vi "Filter_Where.vi"(11 "Filter In":T1[](array[typedef])) -> (3 "WHERE?":string)   [LabVIEW 2020]
uses:
  Controls/Filter.ctl
  Controls/Comparator.ctl
panel:
  out "Array":string[](array[string])
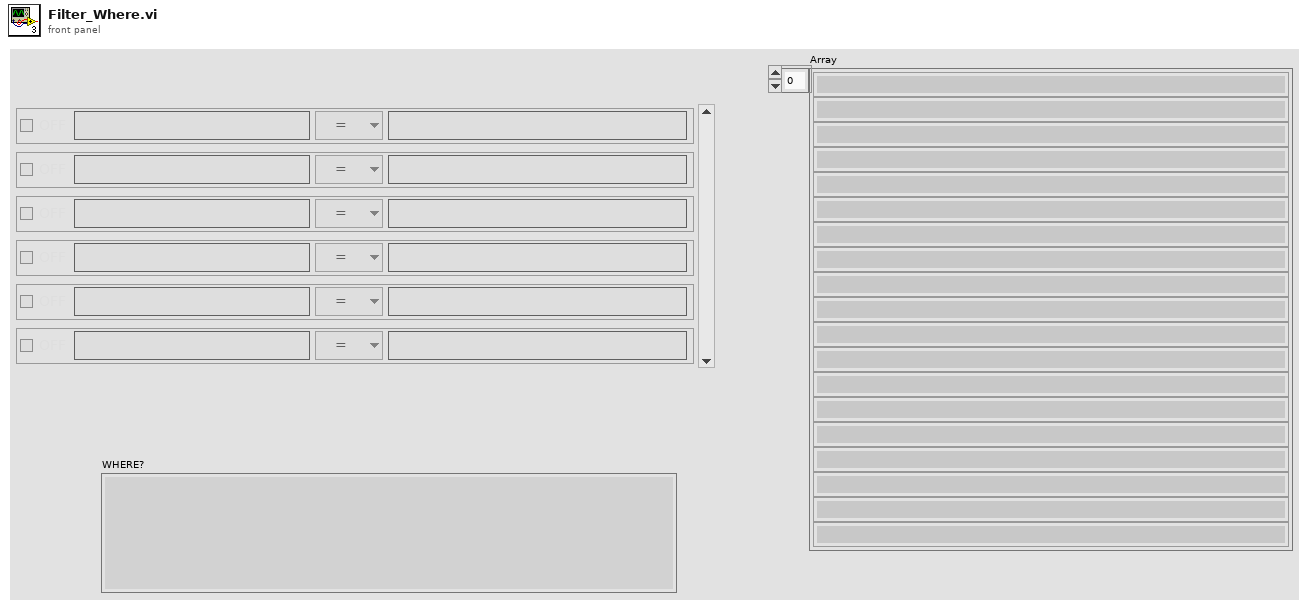
[diagram p1: front panel]
types:
  T1 = typedef "Filter.ctl" = cluster{"Select":bool, "Column":string, "Compare":T2, "Data":string}
  T2 = typedef "Comparator.ctl" = enum16{"=", "<=", ">=", "<", ">", "Like"}
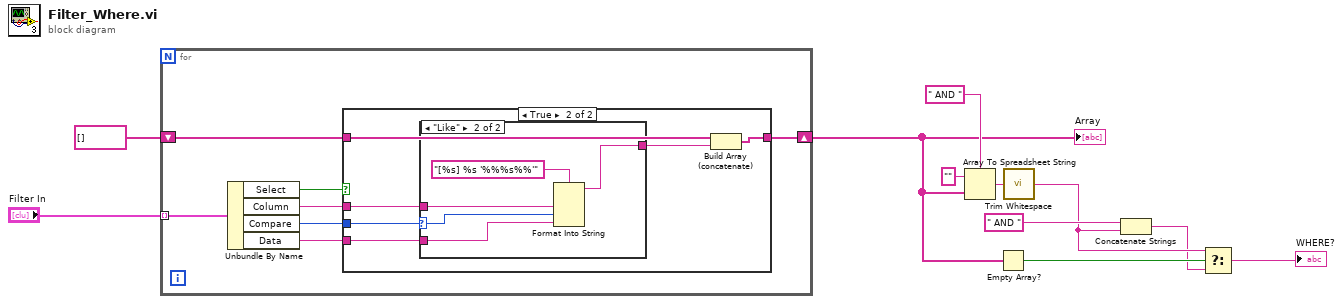
[diagram p0: block diagram]
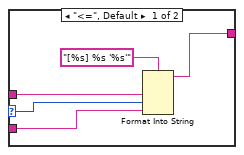
[diagram p3: hidden frame]
diagram:
  n1 = for {
    tunnel: "Filter In" -> [w18] mode=indexing
    shift-right: [w12] -> w6
    shift-left: string[] [] -> [w13]
    n2 = Unbundle By Name(w18) -> ("Select"=w17:bool, "Column"=w16:string, "Compare"=w15:T2, "Data"=w14:string)
    n3 = case shown="True" w17 {
      tunnel: w16 -> [_ w25]
      tunnel: w15 -> [_ w20]
      tunnel: w14 -> [_ w24]
      tunnel: w13 -> [w19 w23]
      tunnel: [w19 w21] -> w12
      frame False {
      }
      frame True {
        n4 = case shown="\"Like\"" w20 {
          selector: w20 -> [w26 w31]
          tunnel: w25 -> [w29 w34]
          tunnel: w24 -> [w28 w33]
          tunnel: [w27 w32] -> w22
          frame "<=", Default {
            n5 = Format Into String(format string="[%s] %s '%s'", w29, w26, w28) -> (resulting string=w27:string)  [unwired: 2 in, 1 out]
          }
          frame "Like" {
            n6 = Format Into String(format string="[%s] %s '%%%s%%'", w34, w31, w33) -> (resulting string=w32:string)  [unwired: 2 in, 1 out]
          }
        }
        n7 = Build Array (concatenate)(w23, w22) -> (w21:string[])
      }
    }
  }
  "Array" <- w6
  n8 = Array To Spreadsheet String(delimiter (Tab)=" AND ", array=w6, 3:"" ("format string")) -> (spreadsheet string=w7:string)
  n9 = Empty Array?(array=w6) -> (empty?=w5:bool)
  n10 = call <vilib>:"Trim Whitespace.vi"("string"=w7) -> ("trimmed string"=w2:string)  [unwired: 1 in]
  n11 = Concatenate Strings(" AND " ("string"), w2) -> (w1:string)
  n12 = Select(t=w2, s=w5, f=w1) -> (s? t:f=→"WHERE?":string)
